vi "Acquisition.vi"(11 "Queue":refnum<queue>) -> ()   [LabVIEW 2013, in "main.lvlib"]
uses:
  main.lvlib
  Controls/Reference AE Control.ctl
  Components/Dependencies.llb/amc_Message Queue.ctl
  Components/Dependencies.llb/amc_Message.ctl
  <vilib>/FTP/util/Keyed Array.ctl
  Controls/Enum Variables.ctl
  Container.vi
  Acquisition/AcqDataQSM.vi
  Control Module/MainControl.vi
  Components/Dependencies.llb/TLB_Dependencies.lvlib
  <vilib>/FTP/NI_FTP.lvlib
panel:
  in  "SegmentCombo":string(combo)
  in  "SegmentAcqString":string="TEXT"
  in  "RingActGraph":u16(ring) caption="Aktive grafer" items=["Begge", "Blå", "Rød"]
  in  "DeflateBtn":bool
  in  "Slide":ext(slide) scale=0.0..300.0
  in  "Stop":bool
  in  "OffsetCalibrationBtn":bool
  in  "Acquisition Btn":bool
  in  "ActivateReservoirBtn":bool
  in  "EmptyReservoirBtn":bool
  in  "PressuriseBtn":bool
  in  "RegulationBtn":bool
  out "Temp":dbl caption="T"
  out "Tank":dbl(slide) scale=0.0..300.0
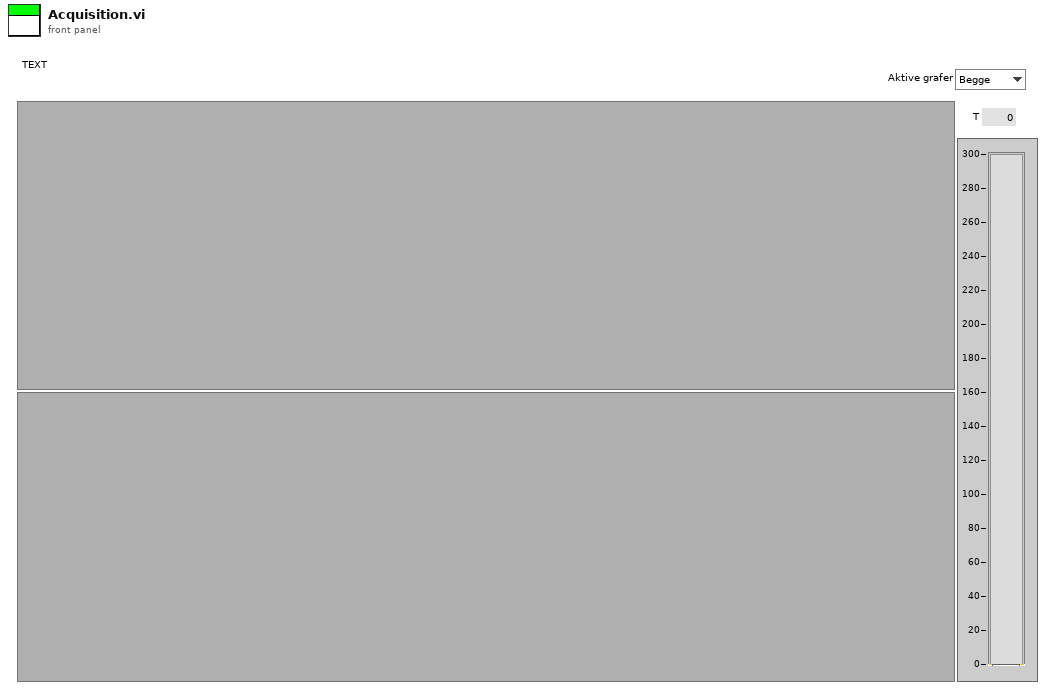
[diagram p1: front panel]
types:
  T1 = typedef "main.lvlib/TLB_Dependencies.lvlib/amc_Message Queue.ctl" = refnum<queue>
  T2 = cluster{"Lower Notifier":refnum<notifier>, "Upper Notifier":refnum<notifier>, "Acquisition Queue":refnum<queue>, "Control Queue":refnum<queue>, "SignalCluster":cluster{"Pump":bool, "Finger":bool, "Ankle":bool, "Fast Def":bool, "Slow Def":bool, "Init Cal":bool, "Table Pres":bool, "Table":bool}, "Segment":string, "Caller Queue":T1, "Control?":bool, "DAQ Active?":bool}
  T3 = typedef "main.lvlib/Reference AE Control.ctl" = enum16{"Initialize", "Set Menu", "Set Profile", "Set Configuration", "Set Configuration_old", "Set Configuration_new", "Set Configuration Method", "Set Acquisition", "Set Data", "Set Journal", "Get"}
  T4 = cluster{"SegmentAcqString":refnum<vi>, "RingActGraph":refnum<vi>}
  T5 = typedef "main.lvlib/Enum Variables.ctl" = enum16{"SetAcqFilter", "GetAcqFilter", "Set Filter", "Get Filter", "Set Height", "Get Height", "Set Recorded Height", "Get Recorded Height", "Set Blue Pressure", "Get Blue Pressure", "Set Red Pressure", "Get Red Pressure", "Init", "Reset Pressure", "Set Red Cursors", "Get Red Cursors", "Set Blue Cursors", "Get Blue Cursors", "Set Language", "Get Language", "Set Active Graphs", "Get ActiveGraphs", "Set Method", "Get Method", "Set Encryption", "Get Encryption", "Set ExcelVersion", "Get ExcelVersion", "Set DICOM Avail", "Get DICOM Avail", "Set DICOM Encode", "Get DICOM Encode", "Set JournalExport", "Get JournalExport", "Set Sequence", "Get Sequence", "Set DAQ Connected", "Get DAQ Connected", "Set Current Graph", "Get Current Graph", "Set General Settings", "Get Hyphenation", "Set Arm Calc Method", "Get Arm Calc Method", "Set Dicom Tags", "Get Dicom Tags", "Set BT Serial", "Get BT Serial", "Set BT Accepted Serials", "Get BT Accepted Serials", "Get BT License", "Set BT License"}
  T6 = cluster{"Pump":bool, "Finger":bool, "Ankle":bool, "Fast Def":bool, "Slow Def":bool, "Init Cal":bool, "Table Pres":bool, "Table":bool}
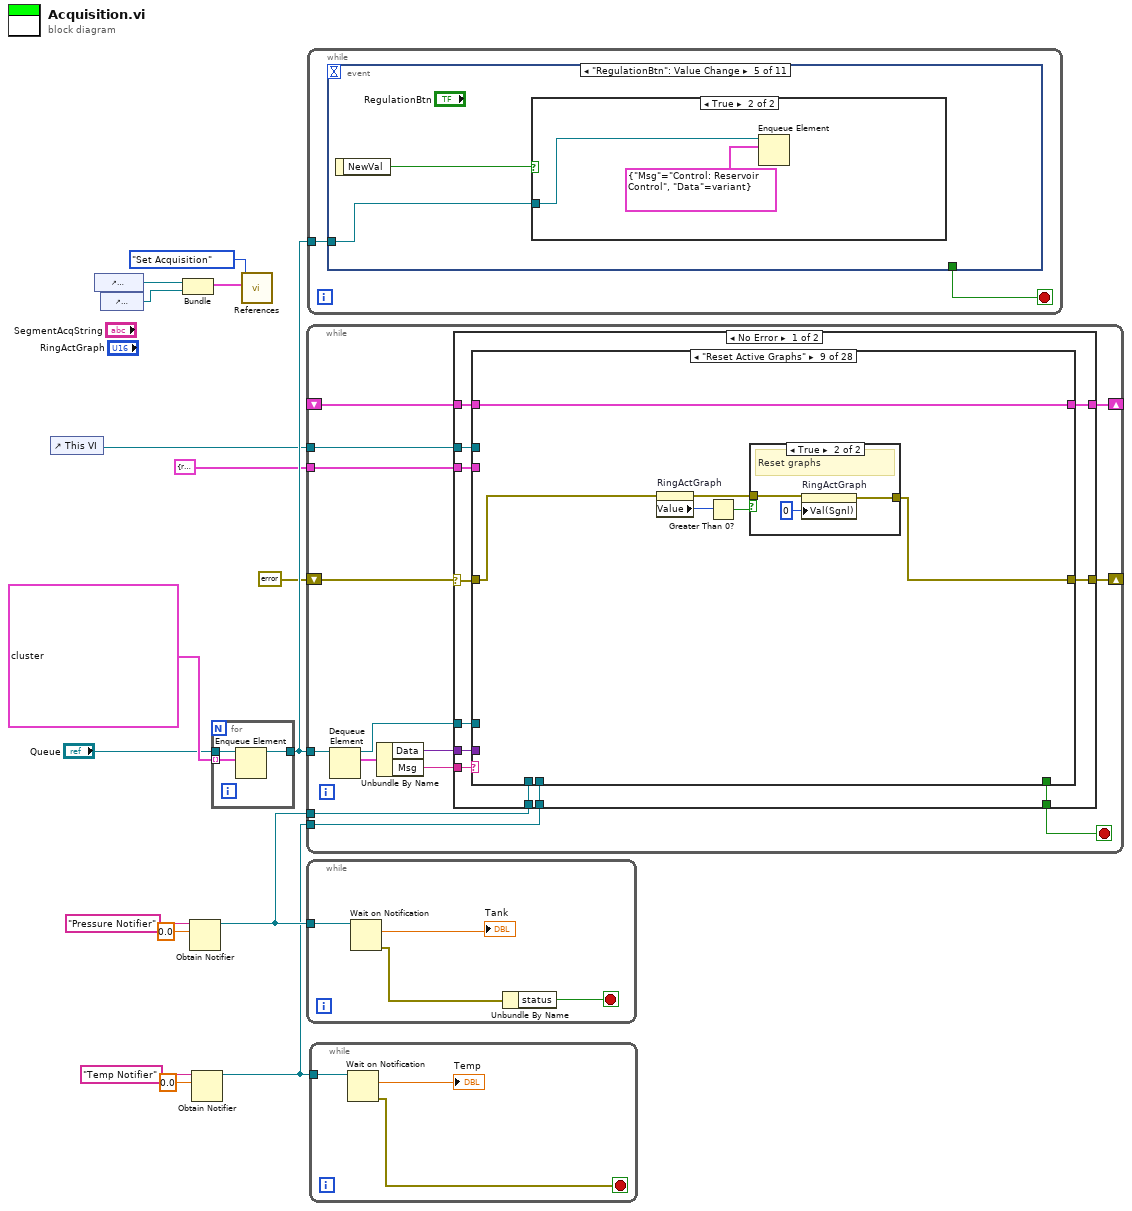
[diagram p0: block diagram]
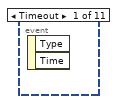
[diagram p2: hidden frame]
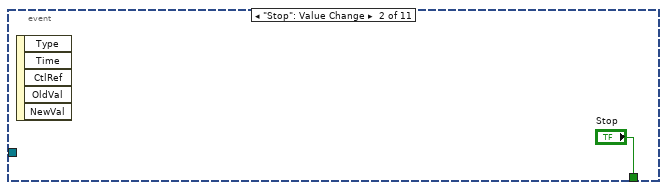
[diagram p3: hidden frame]
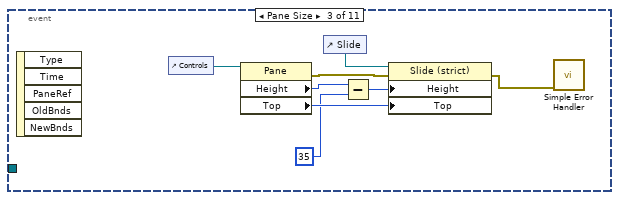
[diagram p4: hidden frame]
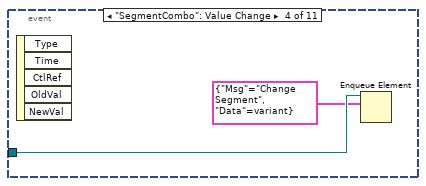
[diagram p5: hidden frame]
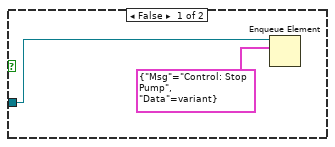
[diagram p6: hidden frame]
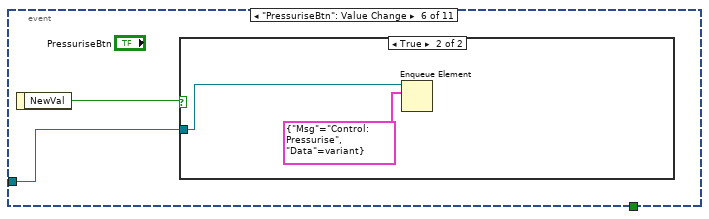
[diagram p7: hidden frame]
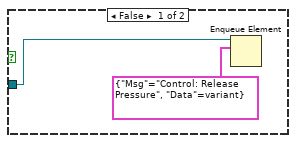
[diagram p8: hidden frame]
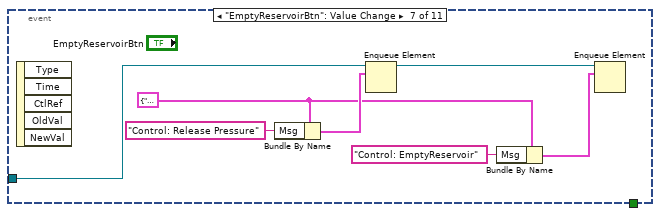
[diagram p9: hidden frame]
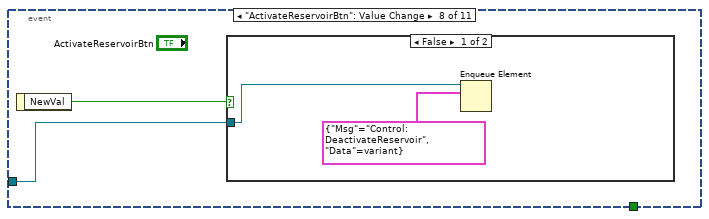
[diagram p10: hidden frame]
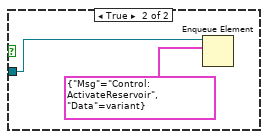
[diagram p11: hidden frame]
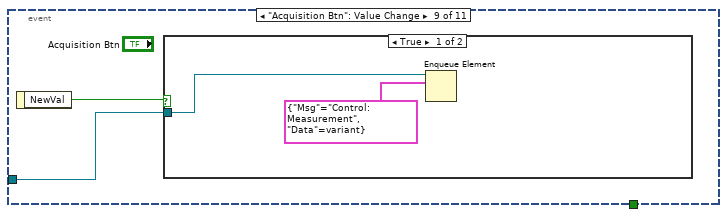
[diagram p12: hidden frame]
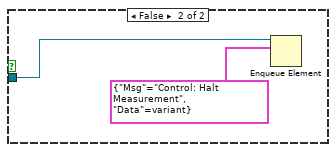
[diagram p13: hidden frame]
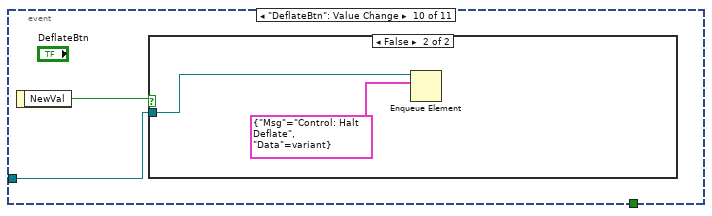
[diagram p14: hidden frame]
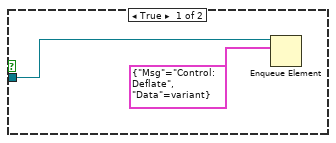
[diagram p15: hidden frame]
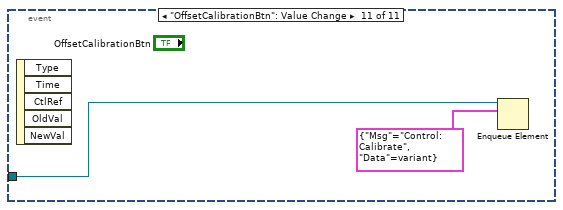
[diagram p16: hidden frame]
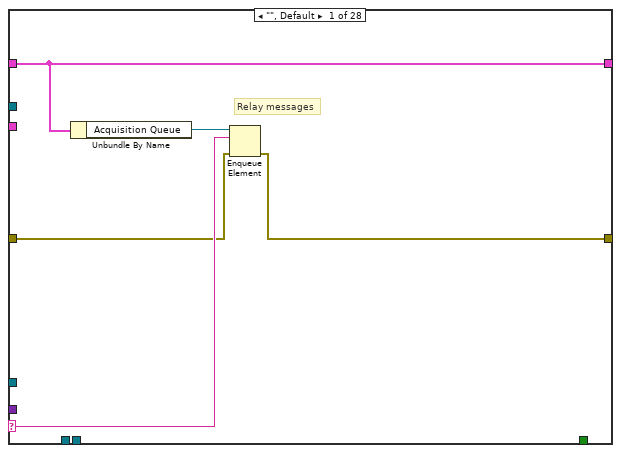
[diagram p17: hidden frame]
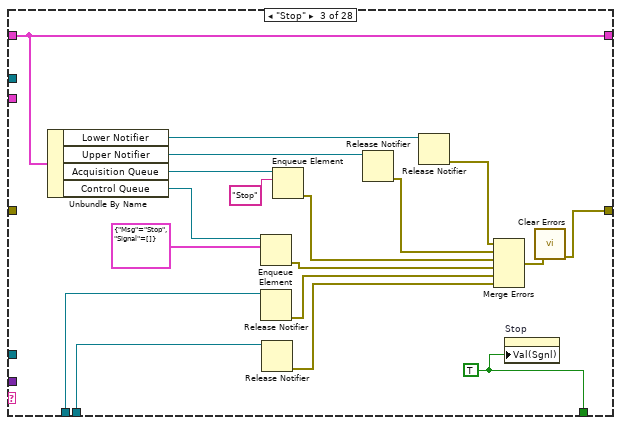
[diagram p19: hidden frame]
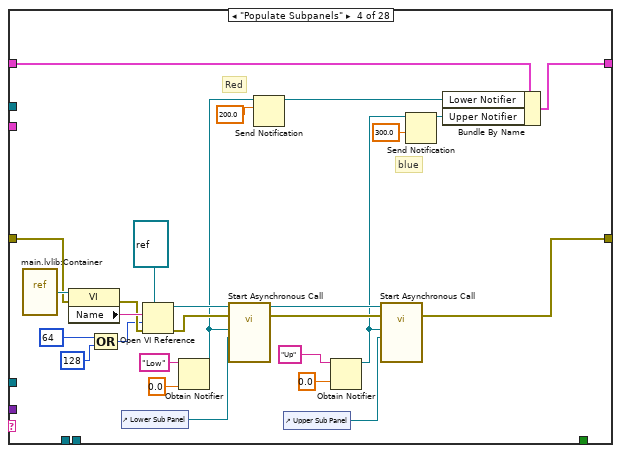
[diagram p20: hidden frame]
diagram:
  n1 = control-ref of="This VI"() -> (w5:refnum<vi>)
  n2 = control-ref of="SegmentAcqString"() -> (w16:refnum<vi>)
  n3 = control-ref of="RingActGraph"() -> (w15:refnum<vi>)
  n4 = Bundle("SegmentAcqString"=w16, "RingActGraph"=w15) -> (w14:T4)  [unwired: 1 in]
  n5 = Obtain Notifier(name (unnamed)="Pressure Notifier", notification data type=0.0) -> (notifier out=w9:refnum<notifier>)  [unwired: 2 in, 2 out]
  n6 = Obtain Notifier(name (unnamed)="Temp Notifier", notification data type=0.0) -> (notifier out=w1:refnum<notifier>)  [unwired: 2 in, 2 out]
  n7 = for {
    tunnel: "Queue" -> [w17]
    tunnel: [w19] -> w11
    tunnel: cluster{"Msg":string, "Data":variant}[] [{"Msg"="Init", "Data"=variant}, {"Msg"="Populate Subpanels", "Data"=variant}] -> [w18] mode=indexing
    n8 = Enqueue Element(queue=w17, element=w18) -> (queue out=w19:refnum<queue>)  [unwired: 2 in, 2 out]
  }
  n9 = call "References.vi"("variant"=w14, "Reference AE Control"=Reference_AE_Control."Set Acquisition") -> ()  [unwired: 8 in, 2 out]
  n10 = while {
    tunnel: w11 -> [w33]
    shift-right: [w30] -> _
    shift-left: _ -> [w29]
    tunnel: w9 -> [w27]
    tunnel: T2 {"Lower Notifier"=refnum, "Upper Notifier"=refnum, "Acquisition Queue"=refnum, "Control Queue"=refnum, "SignalCluster"={"Pump"=TRUE, "Finger"=TRUE, "Ankle"=TRUE, "Fast Def"=TRUE, "Slow Def"=TRUE, "Init Cal"=TRUE, "Table Pres"=TRUE, "Table"=TRUE}, "Segment"="", "Caller Queue"=refnum, "Control?"=TRUE, "DAQ Active?"=TRUE} -> [w26]
    shift-right: [w24] -> _
    shift-left: errorcluster {"status"=FALSE, "code"=0, "source"=""} ("error out") -> [w23]
    tunnel: w5 -> [w21]
    tunnel: w1 -> [w20]
    stop <- w31 stop-if-true
    n11 = Dequeue Element(queue=w33) -> (queue out=w25:refnum<queue>, element=w32:cluster{"Msg":string, "Data":variant})  [unwired: 2 in, 2 out]
    n12 = Unbundle By Name(w32) -> ("Data"=w28:variant, "Msg"=w22:string)
    n13 = case shown="No Error" w23 {
      selector: w23 -> [w36 w319]
      tunnel: w22 -> [w45 _]
      tunnel: [w44 w317] -> w31
      tunnel: [w43 w323] -> w30
      tunnel: w29 -> [w42 w323]
      tunnel: w28 -> [w41 _]
      tunnel: w27 -> [w40 _]
      tunnel: w26 -> [w39 _]
      tunnel: w25 -> [w38 w322]
      tunnel: [w37 errorcluster {"status"=FALSE, "code"=0, "source"=""} ("error out")] -> w24
      tunnel: w21 -> [w35 _]
      tunnel: w20 -> [w34 _]
      frame No Error {
        n14 = case shown="\"Reset Active Graphs\"" w45 {
          selector: w45 -> [w48 _ _ _ _ _ _ _ _ _ _ _ _ _ _ _ _ _ _ _ _ _ _ _ _ _ _ _]
          tunnel: [_ _ w67 _ _ _ _ _ _ _ _ _ _ _ _ _ _ _ _ _ _ _ _ _ _ _ _ _] -> w44
          tunnel: [w50 w52 w70 w90 w101 w111 w121 w128 w134 w139 w152 w169 w189 w206 w223 w228 w231 w236 w244 w248 w258 w264 w271 w277 w289 w298 w305 w316] -> w43
          tunnel: w42 -> [w50 _ w70 w91 w102 w111 w120 w127 w134 w139 w151 w170 w190 w207 w223 w228 w231 w236 w245 w249 w258 w265 w272 w278 w290 w299 w306 w316]
          tunnel: w41 -> [_ _ _ _ w105 w112 w119 w124 _ w144 _ _ _ _ _ _ _ _ _ _ _ _ _ _ _ _ _ _]
          tunnel: w40 -> [_ _ w66 _ _ _ _ _ _ _ _ w161 _ w209 _ _ _ _ _ _ _ _ _ _ _ _ _ _]
          tunnel: w39 -> [_ w52 _ _ _ _ _ _ _ _ _ _ _ _ _ _ _ _ _ _ _ _ _ _ _ _ _ _]
          tunnel: w38 -> [_ _ _ _ _ _ _ _ _ _ _ w159 _ _ _ _ _ _ _ _ _ _ _ _ _ _ _ _]
          tunnel: [w46 w51 w55 w80 w98 w108 w115 w122 w129 w145 w146 w154 w187 w204 w219 w224 w229 w233 w237 w246 w254 w259 w266 w274 w285 w296 w303 w309] -> w37
          tunnel: w36 -> [w47 w51 _ w88 w99 w109 w116 w123 w131 w143 w147 w156 w184 w203 w220 w225 w230 w234 w239 w247 w255 w260 w267 w275 w286 w295 w302 w310]
          tunnel: w35 -> [_ _ _ _ _ _ _ _ _ _ _ _ _ _ _ _ _ _ _ _ _ _ _ _ _ _ _ _]
          tunnel: w34 -> [_ _ w54 _ _ _ _ _ _ _ _ w153 _ _ _ _ _ _ _ _ _ _ _ _ _ _ _ _]
          frame "", Default {
            # "Relay messages"
            n15 = Unbundle By Name(w50) -> ("Acquisition Queue"=w49:refnum<queue>)
            n16 = Enqueue Element(queue=w49, element=w48, error in (no error)=w47) -> (error out=w46:errorcluster)  [unwired: 1 in, 2 out]
          }
          frame "Init" {
          }
          frame "Stop" {
            w67 = TRUE
            n17 = Unbundle By Name(w70) -> ("Lower Notifier"=w69:refnum<notifier>, "Upper Notifier"=w68:refnum<notifier>, "Acquisition Queue"=w61:refnum<queue>, "Control Queue"=w60:refnum<queue>)
            n18 = Enqueue Element(queue=w60, element=cluster{"Msg":string, "Signal":bool[]} {"Msg"="Stop", "Signal"=[]}) -> (error out=w56:errorcluster)  [unwired: 2 in, 2 out]
            n19 = Release Notifier(notifier=w66) -> (error out=w62:errorcluster)  [unwired: 2 in, 2 out]
            n20 = Release Notifier(notifier=w54) -> (error out=w53:errorcluster)  [unwired: 2 in, 2 out]
            n21 = Enqueue Element(queue=w61, element="Stop") -> (error out=w57:errorcluster)  [unwired: 2 in, 2 out]
            n22 = Release Notifier(notifier=w68) -> (error out=w63:errorcluster)  [unwired: 2 in, 2 out]
            n23 = Release Notifier(notifier=w69) -> (error out=w64:errorcluster)  [unwired: 2 in, 2 out]
            n24 = Merge Errors(w64, w63, w57, w56, w62, w53) -> (w65:errorcluster)
            n25 = property on="Stop" class="Bool (strict)"("Val(Sgnl)"=w67) -> ()  [unwired: 2 in, 2 out]
            n26 = call <vilib>:"Clear Errors.vi"("error in (no error)"=w65) -> ("error out"=w55:errorcluster)  [unwired: 6 in]
          }
          frame "Populate Subpanels" {
            # "blue"
            # "Red"
            n27 = vi-ref "main.lvlib:Container.vi"() -> (w97:refnum<vi>)
            n28 = property class="VI"(reference=w97, error in=w88) -> (error out=w92:errorcluster, "Name"=w96:string)  [unwired: 1 out]
            n29 = Compound Arithmetic op=OR(64, 128) -> (w85:i32)
            n30 = control-ref of="Lower Sub Panel"() -> (w82:refnum<vi>)
            n31 = Open VI Reference(type specifier VI Refnum (for type only)=refnum<vi> refnum, vi path=w96, options=w85, error in (no error)=w92) -> (vi reference=w94:refnum<vi>, error out=w93:errorcluster)  [unwired: 2 in]
            n32 = Obtain Notifier(name (unnamed)="Low", notification data type=0.0) -> (notifier out=w76:refnum<notifier>)  [unwired: 2 in, 2 out]
            n33 = call-by-ref "Start Asynchronous Call"(reference=w94, error in=w93, "SubPnl Refnum"=w82, "Notifier"=w76) -> (reference out=w83:refnum<vi>, error out=w79:errorcluster)  [unwired: 10 in]
            n34 = Send Notification(notification=200.0, notifier=w76) -> (notifier out=w75:refnum<notifier>)  [unwired: 1 in, 1 out]
            n35 = control-ref of="Upper Sub Panel"() -> (w81:refnum<vi>)
            n36 = Obtain Notifier(name (unnamed)="Up", notification data type=0.0) -> (notifier out=w72:refnum<notifier>)  [unwired: 2 in, 2 out]
            n37 = call-by-ref "Start Asynchronous Call"(reference=w83, error in=w79, "SubPnl Refnum"=w81, "Notifier"=w72) -> (error out=w80:errorcluster)  [unwired: 10 in, 1 out]
            n38 = Send Notification(notification=300.0, notifier=w72) -> (notifier out=w73:refnum<notifier>)  [unwired: 1 in, 1 out]
            n39 = Bundle By Name(cluster=w91, "Lower Notifier"=w75, "Upper Notifier"=w73) -> (w90:T2)
          }
          frame "Set Mode" {
            n40 = Variant To Data(type=FALSE, Variant=w105) -> (data=w100:bool)  [unwired: 1 in, 1 out]
            n41 = case shown="True" w100 {
              tunnel: [1 230] -> w103
              frame False {
              }
              frame True {
              }
            }
            n42 = Bundle By Name(cluster=w102, "Control?"=w100) -> (w101:T2)
            n43 = property on="Splitter 3" class="Splitter"(error in=w99, "Position"=w103) -> (error out=w98:errorcluster)  [unwired: 1 in, 1 out]
          }
          frame "Set Color" {
            n44 = control-ref of="This VI"() -> (w110:refnum<vi>)
            n45 = Variant To Data(error in=w109, type=u32 0 ("Pane Color"), Variant=w112) -> (data=w113:u32, error out=w108:errorcluster)
            n46 = call "Set VI Color.vi"("Pane Color"=w113, "VI in"=w110) -> ()  [unwired: 10 in]
          }
          frame "Set Caller Queue" {
            n47 = Unbundle By Name(w120) -> ("Caller Queue"=w118:T1)
            n48 = Variant To Data(error in=w116, type=w118, Variant=w119) -> (data=w117:T1, error out=w115:errorcluster)
            n49 = Bundle By Name(cluster=w120, "Caller Queue"=w117) -> (w121:T2)
          }
          frame "Set Segment" {
            n50 = Unbundle By Name(w127) -> ("Segment"=w125:string)
            n51 = Variant To Data(error in=w123, type=w125, Variant=w124) -> (data=w126:string, error out=w122:errorcluster)
            n52 = Bundle By Name(cluster=w127, "Segment"=w126) -> (w128:T2)
          }
          frame "Reset Active Graphs" {
            n53 = property on="RingActGraph" class="Ring (strict)"(error in=w131) -> (error out=w130:errorcluster, "Value"=w133:u16)  [unwired: 1 in, 1 out]
            n54 = Greater Than 0?(x=w133) -> (x > 0?=w132:bool)
            n55 = case shown="True" w132 {
              tunnel: w130 -> [w135 w137]
              tunnel: [w135 w136] -> w129
              frame False {
              }
              frame True {
                # "Reset graphs"
                n56 = property on="RingActGraph" class="Ring (strict)"(error in=w137, "Val(Sgnl)"=u16 0 ("Value (Signaling)")) -> (error out=w136:errorcluster)  [unwired: 1 in, 1 out]
              }
            }
          }
          frame "Set Slide" {
            n57 = Variant To Data(error in=w143, type=0.0, Variant=w144) -> (data=w140:dbl, error out=w142:errorcluster)
            n58 = property on="Slide" class="Slide (strict)"(error in=w142, "Val(Sgnl)"=w140) -> (error out=w145:errorcluster)  [unwired: 1 in, 1 out]
          }
          frame "Change Segment" {
            n59 = Unbundle By Name(w151) -> ("Caller Queue"=w150:T1)
            n60 = call "AMC Send Local Message.vi"("error in (no error)"=w147, "Message Value"="SegmentCombo", "Message Name"="Change Segment", "Message Queue in"=w150) -> ("error out"=w146:errorcluster)  [unwired: 6 in, 1 out]
            n61 = Bundle By Name(cluster=w151, "Segment"="SegmentCombo") -> (w152:T2)
          }
          frame "Initialize DAQ" {
            n62 = vi-ref "main.lvlib:AcqDataQSM.vi"() -> (w178:refnum<vi>)
            n63 = Unbundle By Name(w170) -> ("Upper Notifier"=w174:refnum<notifier>, "Lower Notifier"=w173:refnum<notifier>, "Control?"=w160:bool)
            n64 = property class="VI"(reference=w178, error in=w156) -> (error out=w163:errorcluster, "Name"=w177:string)  [unwired: 1 out]
            n65 = Obtain Queue(element data type="") -> (queue out=w168:refnum<queue>)  [unwired: 4 in, 2 out]
            n66 = Open VI Reference(type specifier VI Refnum (for type only)=refnum<vi> refnum, vi path=w177, options=128, error in (no error)=w163) -> (vi reference=w175:refnum<vi>, error out=w162:errorcluster)  [unwired: 2 in]
            n67 = call-by-ref "Start Asynchronous Call"(reference=w175, error in=w162, "Temp Notifier"=w153, "Pressure Notifier"=w161, "Lower Notifier"=w173, "Upper Notifier"=w174, "Acquisition Control"=w168) -> (reference out=w166:refnum<vi>, error out=w167:errorcluster)  [unwired: 7 in]
            n68 = Close Reference(reference=w166, error in (no error)=w167) -> (error out=w157:errorcluster)
            n69 = Bundle By Name(cluster=w170, "Acquisition Queue"=w168, "DAQ Active?"=TRUE) -> (w169:T2)
            n70 = call "AE Variables.vi"("VariantIn"=TRUE, "error in (no error)"=w157, "Action"=Enum_Variables."Set DAQ Connected") -> ("error out"=w155:errorcluster)  [unwired: 9 in, 7 out]
            n71 = case shown="True" w160 {
              tunnel: w159 -> [_ w183]
              tunnel: [w179 w181] -> w154
              tunnel: w155 -> [w179 w180]
              frame False {
              }
              frame True {
                n72 = Enqueue Element(queue=w183, element=cluster{"Msg":string, "Data":variant} {"Msg"="Initialize Control", "Data"=variant}, error in (no error)=w180) -> (error out=w181:errorcluster)  [unwired: 1 in, 2 out]
              }
            }
          }
          frame "Halt DAQ" {
            # "Queues are destroyed in subvi"
            n73 = Unbundle By Name(w190) -> ("Acquisition Queue"=w196:refnum<queue>, "Control Queue"=w191:refnum<queue>, "Control?"=w192:bool)
            n74 = Enqueue Element(queue=w196, element="Stop", error in (no error)=w184) -> (error out=w185:errorcluster)  [unwired: 1 in, 2 out]
            n75 = case shown="True" w192 {
              tunnel: w191 -> [_ w198]
              tunnel: [w197 w200] -> w186
              tunnel: w185 -> [w197 w199]
              frame False {
              }
              frame True {
                n76 = Enqueue Element(queue=w198, element=cluster{"Msg":string, "Signal":bool[]} {"Msg"="Stop", "Signal"=[]}, error in (no error)=w199) -> (error out=w200:errorcluster)  [unwired: 1 in, 2 out]
              }
            }
            n77 = Bundle By Name(cluster=w190, "DAQ Active?"=FALSE) -> (w189:T2)
            n78 = call "AE Variables.vi"("VariantIn"=FALSE, "error in (no error)"=w186, "Action"=Enum_Variables."Set DAQ Connected") -> ("error out"=w187:errorcluster)  [unwired: 9 in, 7 out]
          }
          frame "Initialize Control" {
            n79 = vi-ref "main.lvlib:MainControl.vi"() -> (w218:refnum<vi>)
            n80 = Obtain Queue(element data type=cluster{"Msg":string, "Signal":bool[]} {"Msg"="", "Signal"=[]}) -> (queue out=w205:refnum<queue>)  [unwired: 4 in, 2 out]
            n81 = property class="VI"(reference=w218, error in=w203) -> (error out=w211:errorcluster, "Name"=w217:string)  [unwired: 1 out]
            n82 = control-ref of="Slide"() -> (w202:refnum<vi>)
            n83 = Open VI Reference(type specifier VI Refnum (for type only)=refnum<vi> refnum, vi path=w217, options=128, error in (no error)=w211) -> (vi reference=w215:refnum<vi>, error out=w210:errorcluster)  [unwired: 2 in]
            n84 = call-by-ref "Start Asynchronous Call"(reference=w215, error in=w210, "Slide"=w202, "notifier in"=w209, "queue in"=w205) -> (reference out=w212:refnum<vi>, error out=w213:errorcluster)  [unwired: 9 in]
            n85 = Close Reference(reference=w212, error in (no error)=w213) -> (error out=w204:errorcluster)
            n86 = Bundle By Name(cluster=w207, "Control Queue"=w205) -> (w206:T2)
          }
          frame "Control: Automatic" {
            n87 = Unbundle By Name(w223) -> ("Control Queue"=w222:refnum<queue>, "Segment"=w221:string)
            n88 = call "Start Automatic Execution.vi"("error in (no error)"=w220, "Measuring Limb"=w221, "Queue in"=w222) -> ("error out"=w219:errorcluster)  [unwired: 8 in]
          }
          frame "Control: Stop Pump" {
            n89 = Unbundle By Name(w228) -> ("Control Queue"=w227:refnum<queue>, "SignalCluster"=w226:T6)
            n90 = call "Stop Pump.vi"("error in (no error)"=w225, "SignalCluster"=w226, "Queue in"=w227) -> ("error out"=w224:errorcluster)  [unwired: 8 in]
          }
          frame "Control: Reservoir Control" {
            n91 = Unbundle By Name(w231) -> ("Control Queue"=w232:refnum<queue>)
            n92 = call "ReservoirControl.vi"("error in (no error)"=w230, "Queue in"=w232) -> ("error out"=w229:errorcluster)  [unwired: 9 in]
          }
          frame "Control: Regulation Stopped" {
            n93 = property on="RegulationBtn" class="Bool (strict)"(error in=w234, "Value"=FALSE ("RegulationBtn")) -> (error out=w233:errorcluster)  [unwired: 1 in, 1 out]
          }
          frame "Control: Release Pressure" {
            n94 = Unbundle By Name(w245) -> ("Control Queue"=w242:refnum<queue>, "SignalCluster"=w241:T6)
            n95 = call "Release Pressure.vi"("error in (no error)"=w239, "SignalCluster in"=w241, "Queue in"=w242) -> ("error out"=w238:errorcluster, "SignalCluster out"=w243:T6)  [unwired: 7 in]
            n96 = Bundle By Name(cluster=w245, "SignalCluster"=w243) -> (w244:T2)
            n97 = property on="PressuriseBtn" class="Bool (strict)"(error in=w238, "Value"=FALSE ("PressuriseBtn")) -> (error out=w237:errorcluster)  [unwired: 1 in, 1 out]
          }
          frame "Control: Pressurise" {
            n98 = Unbundle By Name(w249) -> ("Control Queue"=w253:refnum<queue>, "SignalCluster"=w252:T6, "Segment"=w251:string)
            n99 = call "Pressurise.vi"("error in (no error)"=w247, "Measuring Limb"=w251, "SignalCluster in"=w252, "Queue in"=w253) -> ("error out"=w246:errorcluster, "SignalCluster out"=w250:T6)  [unwired: 6 in]
            n100 = Bundle By Name(cluster=w249, "SignalCluster"=w250) -> (w248:T2)
          }
          frame "Control: EmptyReservoir" {
            n101 = Unbundle By Name(w258) -> ("Control Queue"=w257:refnum<queue>, "SignalCluster"=w256:T6)
            n102 = call "Empty Reservoir.vi"("error in (no error)"=w255, "SignalCluster"=w256, "Queue in"=w257) -> ("error out"=w254:errorcluster)  [unwired: 8 in]
          }
          frame "Control: ActivateReservoir" {
            n103 = Unbundle By Name(w265) -> ("Control Queue"=w262:refnum<queue>, "SignalCluster"=w261:T6)
            n104 = call "Activate Reservoir.vi"("error in (no error)"=w260, "SignalCluster in"=w261, "Queue in"=w262) -> ("error out"=w259:errorcluster, "SignalCluster out"=w263:T6)  [unwired: 7 in]
            n105 = Bundle By Name(cluster=w265, "SignalCluster"=w263) -> (w264:T2)
          }
          frame "Control: DeactivateReservoir" {
            n106 = Unbundle By Name(w272) -> ("Control Queue"=w269:refnum<queue>, "SignalCluster"=w268:T6)
            n107 = call "Deactivate Reservoir.vi"("error in (no error)"=w267, "SignalCluster in"=w268, "Queue in"=w269) -> ("error out"=w266:errorcluster, "SignalCluster out"=w270:T6)  [unwired: 7 in]
            n108 = Bundle By Name(cluster=w272, "SignalCluster"=w270) -> (w271:T2)
          }
          frame "Control: Measurement" {
            n109 = Unbundle By Name(w278) -> ("Control Queue"=w280:refnum<queue>, "SignalCluster"=w279:T6, "Caller Queue"=w283:T1)
            n110 = call "AMC Send Local Messages.vi"("error in (no error)"=w275, "Message Names"=string[] ["CreateLogPath", "Acquisition"], "Message Queue in"=w283) -> ("error out"=w281:errorcluster)  [unwired: 7 in, 1 out]
            n111 = call "Deflate.vi"("error in (no error)"=w281, "SignalCluster in"=w279, "Queue in"=w280) -> ("error out"=w274:errorcluster, "SignalCluster out"=w276:T6)  [unwired: 7 in]
            n112 = Bundle By Name(cluster=w278, "SignalCluster"=w276) -> (w277:T2)
            n113 = property on="DeflateBtn" class="Bool (strict)"("Value"=TRUE ("DeflateBtn")) -> ()  [unwired: 2 in, 2 out]
          }
          frame "Control: Halt Measurement" {
            n114 = Unbundle By Name(w290) -> ("Control Queue"=w292:refnum<queue>, "SignalCluster"=w291:T6, "Caller Queue"=w294:T1)
            n115 = call "AMC Send Local Messages.vi"("error in (no error)"=w286, "Message Names"=string[] ["Stop Acquisition", "LogData", "AddTreeItems", "ProcessRecent", "Display Data"], "Message Queue in"=w294) -> ("error out"=w293:errorcluster)  [unwired: 7 in, 1 out]
            n116 = call "Halt Deflate.vi"("error in (no error)"=w293, "SignalCluster in"=w291, "Queue in"=w292) -> ("error out"=w285:errorcluster, "SignalCluster out"=w288:T6)  [unwired: 7 in]
            n117 = Bundle By Name(cluster=w290, "SignalCluster"=w288) -> (w289:T2)
            n118 = property on="DeflateBtn" class="Bool (strict)"("Value"=FALSE ("DeflateBtn")) -> ()  [unwired: 2 in, 2 out]
          }
          frame "Control: Deflate" {
            n119 = Unbundle By Name(w299) -> ("Control Queue"=w301:refnum<queue>, "SignalCluster"=w300:T6)
            n120 = call "Deflate.vi"("error in (no error)"=w295, "SignalCluster in"=w300, "Queue in"=w301) -> ("error out"=w296:errorcluster, "SignalCluster out"=w297:T6)  [unwired: 7 in]
            n121 = Bundle By Name(cluster=w299, "SignalCluster"=w297) -> (w298:T2)
          }
          frame "Control: Halt Deflate" {
            n122 = Unbundle By Name(w306) -> ("Control Queue"=w308:refnum<queue>, "SignalCluster"=w307:T6)
            n123 = call "Halt Deflate.vi"("error in (no error)"=w302, "SignalCluster in"=w307, "Queue in"=w308) -> ("error out"=w303:errorcluster, "SignalCluster out"=w304:T6)  [unwired: 7 in]
            n124 = Bundle By Name(cluster=w306, "SignalCluster"=w304) -> (w305:T2)
          }
          frame "Control: Calibrate" {
            n125 = Unbundle By Name(w316) -> ("Control Queue"=w315:refnum<queue>, "SignalCluster"=w314:T6)
            n126 = call "Initialize Calibration.vi"("error in (no error)"=w310, "SignalCluster"=w314, "Queue in"=w315) -> ("error out"=w311:errorcluster, "SignalCluster out"=w312:T6, "Queue out"=w313:refnum<queue>)  [unwired: 6 in]
            n127 = call "Calibrate.vi"("error in (no error)"=w311, "SignalCluster"=w312, "Queue in"=w313) -> ("error out"=w309:errorcluster)  [unwired: 8 in]
          }
        }
      }
      frame Error {
        # "Need to handle the errors somehow."
        n128 = call <vilib>:"Simple Error Handler.vi"("error in (no error)"=w319) -> ()  [unwired: 4 in, 5 out]
        n129 = Enqueue Element(queue=w322, element=cluster{"Msg":string, "Data":variant} {"Msg"="Stop", "Data"=variant}) -> (error out=w318:errorcluster)  [unwired: 2 in, 2 out]
        n130 = Unbundle By Name(w318) -> ("status"=w317:bool)
      }
    }
  }
  n131 = while {
    tunnel: w9 -> [w327]
    stop <- w325 stop-if-true
    n132 = Wait on Notification(notifier=w327) -> (notification=→"Tank":dbl, error out=w326:errorcluster)  [unwired: 3 in, 2 out]
    n133 = Unbundle By Name(w326) -> ("status"=w325:bool)
  }
  n134 = while {
    tunnel: w11 -> [w328]
    stop <- w329 stop-if-true
    n135 = event shown="[4] \"RegulationBtn\": Value Change" {
      selector: _ -> [_ _ _ _ _ _ _ _ _ _ _]
      dyn-events: _ -> [_ _ _ _ _ _ _ _ _ _ _]
      timeout: _ -> [_ _ _ _ _ _ _ _ _ _ _]
      tunnel: [_ "Stop" _ _ _ _ _ _ _ _ _] -> w329
      tunnel: w328 -> [_ _ _ w340 w341 w347 w359 w360 w366 w372 w378]
      event Timeout {
        n136 = event-data() -> ()  [unwired: 1 in, 2 out]
      }
      event "Stop": Value Change {
        n137 = event-data() -> ()  [unwired: 1 in, 5 out]
      }
      event Pane Size {
        n138 = event-data() -> ()  [unwired: 1 in, 5 out]
        n139 = control-ref of="Controls"() -> (w335:refnum<vi>)
        n140 = property class="Pane"(reference=w335) -> (error out=w333:errorcluster, "Height"=w337:u32, "Top"=w338:i32)  [unwired: 1 in, 1 out]
        n141 = control-ref of="Slide"() -> (w334:refnum<vi>)
        n142 = Subtract(x=w337, y=35) -> (x-y=w336:u32)
        n143 = property class="Slide (strict)"(reference=w334, error in=w333, "Height"=w336, "Top"=w338) -> (error out=w332:errorcluster)  [unwired: 1 out]
        n144 = call <vilib>:"Simple Error Handler.vi"("error in (no error)"=w332) -> ()  [unwired: 4 in, 5 out]
      }
      event "SegmentCombo": Value Change {
        n145 = event-data() -> ()  [unwired: 1 in, 5 out]
        n146 = Enqueue Element(queue=w340, element=cluster{"Msg":string, "Data":variant} {"Msg"="Change Segment", "Data"=variant}) -> ()  [unwired: 2 in, 3 out]
      }
      event "RegulationBtn": Value Change {
        n147 = event-data() -> ("NewVal"=w342:bool)  [unwired: 1 in]
        n148 = case shown="True" w342 {
          tunnel: w341 -> [w343 w346]
          frame False {
            n149 = Enqueue Element(queue=w343, element=cluster{"Msg":string, "Data":variant} {"Msg"="Control: Stop Pump", "Data"=variant}) -> ()  [unwired: 2 in, 3 out]
          }
          frame True {
            n150 = Enqueue Element(queue=w346, element=cluster{"Msg":string, "Data":variant} {"Msg"="Control: Reservoir Control", "Data"=variant}) -> ()  [unwired: 2 in, 3 out]
          }
        }
      }
      event "PressuriseBtn": Value Change {
        n151 = event-data() -> ("NewVal"=w348:bool)  [unwired: 1 in]
        n152 = case shown="True" w348 {
          tunnel: w347 -> [w350 w352]
          frame False {
            n153 = Enqueue Element(queue=w350, element=cluster{"Msg":string, "Data":variant} {"Msg"="Control: Release Pressure", "Data"=variant}) -> ()  [unwired: 2 in, 3 out]
          }
          frame True {
            n154 = Enqueue Element(queue=w352, element=cluster{"Msg":string, "Data":variant} {"Msg"="Control: Pressurise", "Data"=variant}) -> ()  [unwired: 2 in, 3 out]
          }
        }
      }
      event "EmptyReservoirBtn": Value Change {
        w356 = cluster{"Msg":string, "Data":variant} {"Msg"="", "Data"=variant} ("element")
        n155 = event-data() -> ()  [unwired: 1 in, 5 out]
        n156 = Bundle By Name(cluster=w356, "Msg"="Control: Release Pressure") -> (w358:cluster{"Msg":string, "Data":variant})
        n157 = Enqueue Element(queue=w359, element=w358) -> (queue out=w354:refnum<queue>)  [unwired: 2 in, 2 out]
        n158 = Bundle By Name(cluster=w356, "Msg"="Control: EmptyReservoir") -> (w353:cluster{"Msg":string, "Data":variant})
        n159 = Enqueue Element(queue=w354, element=w353) -> ()  [unwired: 2 in, 3 out]
      }
      event "ActivateReservoirBtn": Value Change {
        n160 = event-data() -> ("NewVal"=w361:bool)  [unwired: 1 in]
        n161 = case shown="False" w361 {
          tunnel: w360 -> [w362 w365]
          frame False {
            n162 = Enqueue Element(queue=w362, element=cluster{"Msg":string, "Data":variant} {"Msg"="Control: DeactivateReservoir", "Data"=variant}) -> ()  [unwired: 2 in, 3 out]
          }
          frame True {
            n163 = Enqueue Element(queue=w365, element=cluster{"Msg":string, "Data":variant} {"Msg"="Control: ActivateReservoir", "Data"=variant}) -> ()  [unwired: 2 in, 3 out]
          }
        }
      }
      event "Acquisition Btn": Value Change {
        n164 = event-data() -> ("NewVal"=w367:bool)  [unwired: 1 in]
        n165 = case shown="True" w367 {
          tunnel: w366 -> [w369 w371]
          frame True {
            n166 = Enqueue Element(queue=w369, element=cluster{"Msg":string, "Data":variant} {"Msg"="Control: Measurement", "Data"=variant}) -> ()  [unwired: 2 in, 3 out]
          }
          frame False {
            n167 = Enqueue Element(queue=w371, element=cluster{"Msg":string, "Data":variant} {"Msg"="Control: Halt Measurement", "Data"=variant}) -> ()  [unwired: 2 in, 3 out]
          }
        }
      }
      event "DeflateBtn": Value Change {
        n168 = event-data() -> ("NewVal"=w373:bool)  [unwired: 1 in]
        n169 = case shown="False" w373 {
          tunnel: w372 -> [w375 w377]
          frame True {
            n170 = Enqueue Element(queue=w375, element=cluster{"Msg":string, "Data":variant} {"Msg"="Control: Deflate", "Data"=variant}) -> ()  [unwired: 2 in, 3 out]
          }
          frame False {
            n171 = Enqueue Element(queue=w377, element=cluster{"Msg":string, "Data":variant} {"Msg"="Control: Halt Deflate", "Data"=variant}) -> ()  [unwired: 2 in, 3 out]
          }
        }
      }
      event "OffsetCalibrationBtn": Value Change {
        n172 = event-data() -> ()  [unwired: 1 in, 5 out]
        n173 = Enqueue Element(queue=w378, element=cluster{"Msg":string, "Data":variant} {"Msg"="Control: Calibrate", "Data"=variant}) -> ()  [unwired: 2 in, 3 out]
      }
    }
  }
  n174 = while {
    tunnel: w1 -> [w382]
    stop <- w381 stop-if-true
    n175 = Wait on Notification(notifier=w382) -> (notification=→"Temp":dbl, error out=w381:errorcluster)  [unwired: 3 in, 2 out]
  }
